vi "Action.vi"(8 "DELTAx":dbl, 11 "action":dbl=-0.5520138637989815) -> ()   [LabVIEW 2017]
uses:
  Global.vi
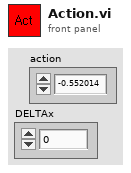
[diagram p1: front panel]
types:
  T1 = typedef "Damping.ctl" = cluster{"Cx":dbl, "Cy":dbl, "Cz":dbl}
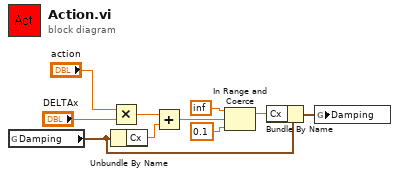
[diagram p0: block diagram]
diagram:
  n1 = global read "Global.vi" "Damping"() -> (w9:T1)
  n2 = Multiply(x="action", y="DELTAx") -> (x*y=w6:dbl)
  n3 = Unbundle By Name(w9) -> ("Cx"=w5:dbl)
  n4 = Add(x=w6, y=w5) -> (x+y=w4:dbl)
  n5 = In Range and Coerce(upper limit=inf, x=w4, lower limit=0.1) -> (coerced(x)=w3:dbl)  [unwired: 1 out]
  n6 = Bundle By Name(cluster=w9, "Cx"=w3) -> (w10:T1)
  n7 = global write "Global.vi" "Damping"(w10) -> ()
